vi "pl1000GetSingle.vi"(8 "error in (no error)":errorcluster, 10 "channel":i32=1, 11 "pl1000 handle":i16) -> (0 "error out":errorcluster, 2 "value":u16, 3 "pl1000 handle out":i16)   [LabVIEW 2010]
doc: "This function returns a single sample value from the specified input channel.\n\nchannel: which channel to sample"
uses:
  pl1000.dll
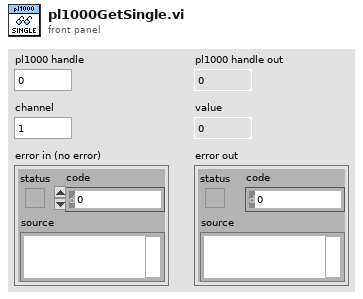
[diagram p1: front panel]
types:
  T1 = cluster{"status":bool, "code":u32, "source":string}
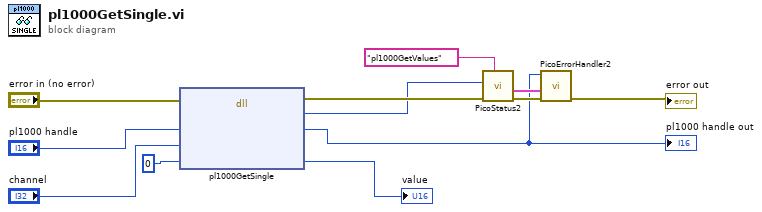
[diagram p0: block diagram]
diagram:
  n1 = dll-call lib="pl1000.dll" fn="pl1000GetSingle"(error in="error in (no error)", "handle"="pl1000 handle", "channel"="channel", "value"=u16 0) -> (error out=w4:errorcluster, "status"=w1:u32, "handle"=w2:i16, "value"=→"value":u16)  [unwired: 3 in, 1 out]
  "pl1000 handle out" <- w2
  n2 = call "PicoStatus2.vi"("PICO source"="pl1000GetValues", "Error in"=w4, "PICO STATUS"=w1) -> ("error out"=w7:errorcluster, "PICO_STATUS out"=w6:T1)  [unwired: 5 in]
  n3 = call "PicoErrorHandler2.vi"("error in (no error)"=w7, "PICO_STATUS in"=w6, "handle In"=w2) -> ("error out"=→"error out":errorcluster)  [unwired: 8 in]
